vi "Initialize.vi"(8 "error in":errorcluster, 9 "Slot Settings":T1, 11 "9226 in":refnum<class "9226.lvclass">) -> (0 "error out":errorcluster, 3 "9226 out":refnum<class "9226.lvclass">)   [LabVIEW 2019, in "Modules.lvlib" / "9226.lvclass"]
uses:
  9226.lvclass
  C:/Users/nitest/Desktop/Git 2019/niveristand-scan-engine-module-libraries/Source/RSI Module/RSI Module.lvclass
  RSI Module/Slot Settings.ctl
  RSI Module/Channels.ctl
  RSI Module/Channel Type.ctl
  RSI Module/Module Models.ctl
  Supported RTD Types.ctl
  9226.lvclass/9226.ctl
  RSI Module/RSI Module.lvclass
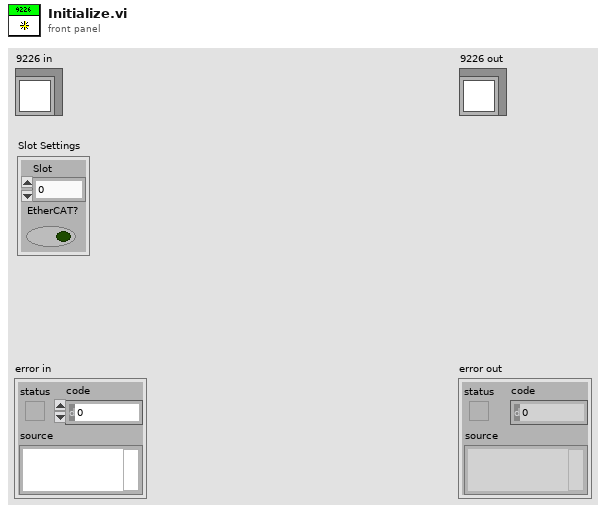
[diagram p1: front panel]
types:
  T1 = typedef "Modules.lvlib/RSI Module.lvclass/Slot Settings.ctl" = cluster{"Slot":u32, "EtherCAT?":bool}
  T2 = typedef "Modules.lvlib/RSI Module.lvclass/Channels.ctl" = cluster{"# Input Channels":i32, "# Output Channels":i32, "Channel Type":T3, "Units":string}
  T3 = typedef "Modules.lvlib/RSI Module.lvclass/Channel Type.ctl" = enum16{"Analog", "Digital"}
  T4 = typedef "Modules.lvlib/9226.lvclass/Supported RTD Types.ctl" = u32
  T5 = cluster{"Ohm degree range":u32, "RTD type":T4, "RTD user-defined A constant":dbl, "RTD user-defined B constant":dbl, "RTD user-defined C constant":dbl, "RTD user-defined Ro constant":dbl}
  T6 = typedef "Modules.lvlib/RSI Module.lvclass/Module Models.ctl" = enum16{"Empty", "NI 9201", "NI 9203", "NI 9205", "NI 9206", "NI 9207", "NI 9208", "NI 9209", "NI 9210", "NI 9211", "NI 9212", "NI 9213", "NI 9214", "NI 9215", "NI 9216", "NI 9217", "NI 9219", "NI 9220", "NI 9221", "NI 9222", "NI 9223", "NI 9224", "NI 9225", "NI 9226", "NI 9227", "NI 9228", "NI 9229", "NI 9233", "NI 9234", "NI 9235", "NI 9236", "NI 9237", "NI 9239", "NI 9242", "NI 9244", "NI 9253", "NI 9263", "NI 9264", "NI 9265", "NI 9266", "NI 9269", "NI 9344", "NI 9350", "NI 9375", "NI 9401", "NI 9402", "NI 9403", "NI 9411", "NI 9421", "NI 9422", "NI 9423", "NI 9425", "NI 9426", "NI 9435", "NI 9436", "NI 9437", "NI 9472", "NI 9474", "NI 9475", "NI 9476", "NI 9477", "NI 9478", "NI 9481", "NI 9482", "NI 9485"}
  T7 = cluster{"Ohm degree range":u32, "RTD type":T4, "RTD user-defined A constant":dbl, "RTD user-defined B constant":dbl, "RTD user-defined C constant":dbl, "RTD user-defined Ro constant":dbl}[]
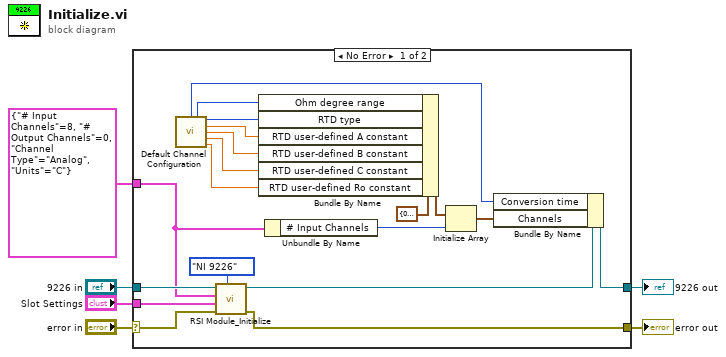
[diagram p0: block diagram]
diagram:
  n1 = case shown="No Error" "error in" {
    selector: "error in" -> [w24 w27]
    tunnel: [w23 w27] -> w3
    tunnel: [w15 w26] -> w5
    tunnel: "Slot Settings" -> [w25 _]
    tunnel: "9226 in" -> [w20 w26]
    tunnel: T2 {"# Input Channels"=8, "# Output Channels"=0, "Channel Type"=enum."Analog", "Units"="C"} ("Channels") -> [w14 _]
    frame No Error {
      n2 = call "Default Channel Configuration.vi"() -> ("Conversion Time"=w13:u32, "Degree Range"=w12:u32, "RTD type"=w11:T4, "RTD_A"=w10:dbl, "RTD_B"=w9:dbl, "RTD_C"=w8:dbl, "RTD_Ro"=w7:dbl)  [unwired: 9 in]
      n3 = call "RSI Module_Initialize.vi"("Module Model"=Module_Models."NI 9226", "error in (no error)"=w24, "Slot Settings"=w25, "Channels"=w14, "RSI Module in"=w20) -> ("error out"=w23:errorcluster, "RSI Module out"=w22:refnum<class "9226.lvclass">)  [unwired: 5 in]
      n4 = Bundle By Name(cluster=T5 {"Ohm degree range"=0, "RTD type"=2, "RTD user-defined A constant"=0.0, "RTD user-defined B constant"=0.0, "RTD user-defined C constant"=0.0, "RTD user-defined Ro constant"=0.0} ("Channel"), "Ohm degree range"=w12, "RTD type"=w11, "RTD user-defined A constant"=w10, "RTD user-defined B constant"=w9, "RTD user-defined C constant"=w8, "RTD user-defined Ro constant"=w7) -> (w18:T5)
      n5 = Unbundle By Name(w14) -> ("# Input Channels"=w17:i32)
      n6 = Initialize Array(w18, w17) -> (w16:T7)
      n7 = Bundle By Name(cluster=w22, "Conversion time"=w13, "Channels"=w16) -> (w15:refnum<class "9226.lvclass">)
    }
    frame Error {
    }
  }
  "error out" <- w3
  "9226 out" <- w5
